vi "Create Lib.vi"(6 "Path":path, 7 "Lib Type":refnum<class "Lib.lvclass">, 8 "error in":errorcluster, 9 "Vis":refnum<class "Vi.lvclass">[](array[class]), 10 "Description":string, 11 "Name":string) -> (0 "error out":errorcluster, 3 "Lib out":refnum<class "Lib.lvclass">)   [LabVIEW 2021, in "TAF Proj Document Type.lvlib" / "Lib.lvclass"]
uses:
  <vilib>/Wovalab/AntiDoc/Document Type/Add-ons/LabVIEW TAF Project/Lib/Lib.lvclass
  C:/Program Files (x86)/National Instruments/LabVIEW 2021/vi.lib/Wovalab/AntiDoc/Bloc/Bloc.lvclass
  <vilib>/Wovalab/AntiDoc/Document Type/Add-ons/LabVIEW TAF Project/Vi/Vi.lvclass
  <vilib>/Wovalab/AntiDoc/Bloc/Bloc.lvclass/Bloc.ctl
  <vilib>/Wovalab/AntiDoc/Document Type/Add-ons/LabVIEW TAF Project/Lib/Lib.lvclass/Lib.ctl
  <vilib>/Wovalab/AntiDoc/Bloc/Write Name.vi
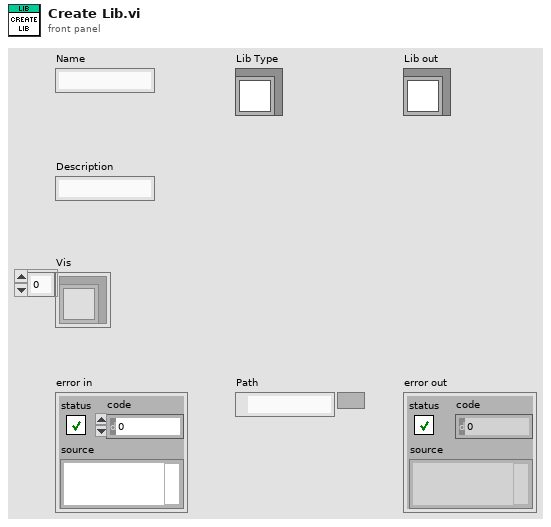
[diagram p1: front panel]
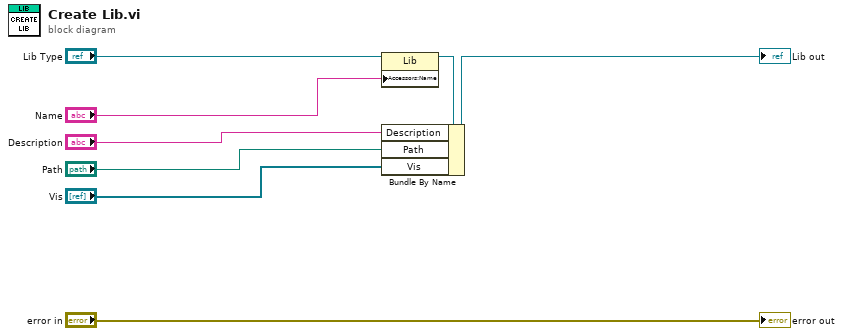
[diagram p0: block diagram]
diagram:
  n1 = property class="Lib"(reference="Lib Type", "Accessors:Name"="Name") -> (reference out=w2:refnum<class "Lib.lvclass">)  [unwired: 1 in, 1 out]
  n2 = Bundle By Name(cluster=w2, "Description"="Description", "Path"="Path", "Vis"="Vis") -> (→"Lib out":refnum<class "Lib.lvclass">)
  "error out" <- "error in"
